vi "Read Analogue.vi"(8 "error in (no error)":errorcluster, 11 "Keysight 5700C in":refnum<class "Keysight 5700C.lvclass">) -> (0 "error out":errorcluster, 2 "Waveforms":waveform(dbl)[](array[waveform]), 3 "Keysight 5700C out":refnum<class "Keysight 5700C.lvclass">)   [LabVIEW 2025, in "Power Supply.lvlib" / "Keysight 5700C.lvclass"]
uses:
  Keysight 5700C.lvclass
  Keysight 5700C.lvclass/Keysight 5700C.ctl
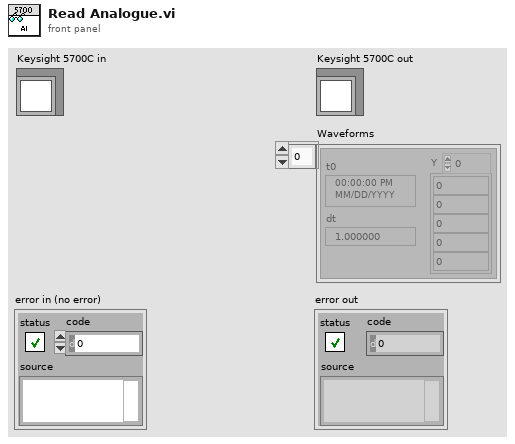
[diagram p1: front panel]
types:
  T1 = typedef "Abstract Engine.lvlibp/Abstract Instrument.lvclass/Channel.ctl" = cluster{"Alias":string, "DataType":enum16{"Anaolg Input", "Waveform"}, "Unit":enum16{"---", "V", "A", "Ohm", "Hz", "uF", "degC", "deg"}, "Upper limit":dbl, "Lower limit":dbl, "Measurement":variant}
  T2 = cluster{"Output Voltage":dbl, "Output Current":dbl}
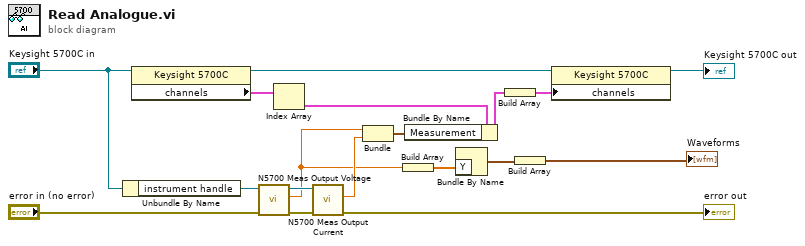
[diagram p0: block diagram]
diagram:
  n1 = Unbundle By Name("Keysight 5700C in") -> ("instrument handle"=w15:refnum<visa-resource-name>)
  n2 = property class="Keysight 5700C"(reference="Keysight 5700C in") -> (reference out=w11:refnum<class "Keysight 5700C.lvclass">, "channels"=w9:T1[])  [unwired: 1 in, 1 out]
  n3 = call <instrlib>:"N5700 Meas Output Voltage.vi"("error"="error in (no error)", "VISA"=w15) -> ("error out"=w14:errorcluster, "Output Voltage"=w4:dbl, "VISA out"=w12:refnum<visa-resource-name>)  [unwired: 4 in]
  n4 = Index Array(array=w9) -> (element=w5:T1)  [unwired: 1 in]
  n5 = call <instrlib>:"N5700 Meas Output Current.vi"("error"=w14, "VISA"=w12) -> ("error out"=→"error out":errorcluster, "Output Current"=w7:dbl)  [unwired: 4 in, 1 out]
  n6 = Bundle("Output Voltage"=w4, "Output Current"=w7) -> (w10:T2)  [unwired: 1 in]
  n7 = Build Array(w4) -> (w3:dbl[])
  n8 = Bundle By Name(cluster=w5, "Measurement"=w10) -> (w8:T1)
  n9 = Bundle By Name("Y"=w3) -> (w2:waveform(dbl))  [unwired: 1 in]
  n10 = Build Array(w8) -> (w6:T1[])
  n11 = Build Array(w2) -> (→"Waveforms":waveform(dbl)[])
  n12 = property class="Keysight 5700C"(reference=w11, "channels"=w6) -> (reference out=→"Keysight 5700C out":refnum<class "Keysight 5700C.lvclass">)  [unwired: 1 in, 1 out]
